vi "CompareStringArrays.vi"(9 "Expected Strings":string[](array[string]), 10 "Actual Strings":string[](array[string])) -> (1 "Message":string, 2 "Equal?":bool)   [LabVIEW 2009, in "UnitTestComparisons.lvlib"]
uses:
  UnitTestComparisons.lvlib
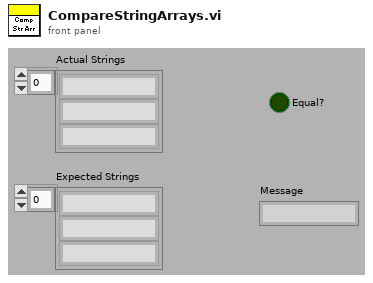
[diagram p1: front panel]
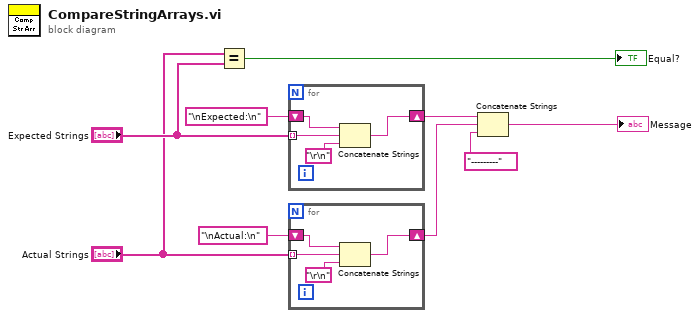
[diagram p0: block diagram]
diagram:
  n1 = Equal?(x="Actual Strings", y="Expected Strings") -> (x = y?=→"Equal?":bool)
  n2 = for {
    tunnel: "Expected Strings" -> [w13] mode=indexing
    shift-right: [w10] -> w6
    shift-left: "\nExpected:\n" ("string") -> [w12]
    n3 = Concatenate Strings(w12, w13, "\r\n") -> (w10:string)
  }
  n4 = for {
    tunnel: "Actual Strings" -> [w17] mode=indexing
    shift-right: [w14] -> w5
    shift-left: "\nActual:\n" ("string") -> [w16]
    n5 = Concatenate Strings(w16, w17, "\r\n") -> (w14:string)
  }
  n6 = Concatenate Strings(w6, w5, "---------" ("string")) -> (→"Message":string)
